vi "make arbitrary waveform_MD.vi"() -> ()   [LabVIEW 2012]
uses:
  Custom Controls/scan mode main settings tab.ctl
  GFG/GFGDisplayRefsGet.vi
  GFG/GFGnumericGet.vi
  GFG/GFGfpRefGet.vi
  GFG/GFGImageRefsGet.vi
  GFG/GFG library.lvlib
  <vilib>/vision/NI_Vision_Development_Module.lvlib
panel:
  out "Source VI":string
  out "error out 3":errorcluster
  out "error out 2":errorcluster
  out "error out":errorcluster
  out "XY Graph 3":cluster{"Y":dbl[], "Y":dbl[]}[](graph)
  out "XY Graph 2":cluster{"Y":dbl[], "Y":dbl[]}[](graph)
  out "XY Graph":cluster{"Y":dbl[], "Y":dbl[]}[](graph)
  out "Waveform Graph 4":dbl[](graph)
  out "Waveform Graph 3":dbl[](graph)
  out "Waveform Graph 2":waveform(dbl)(graph)
  out "Waveform Graph":waveform(dbl)(graph)
  out "size(s) 2":i32
  out "size(s)":i32
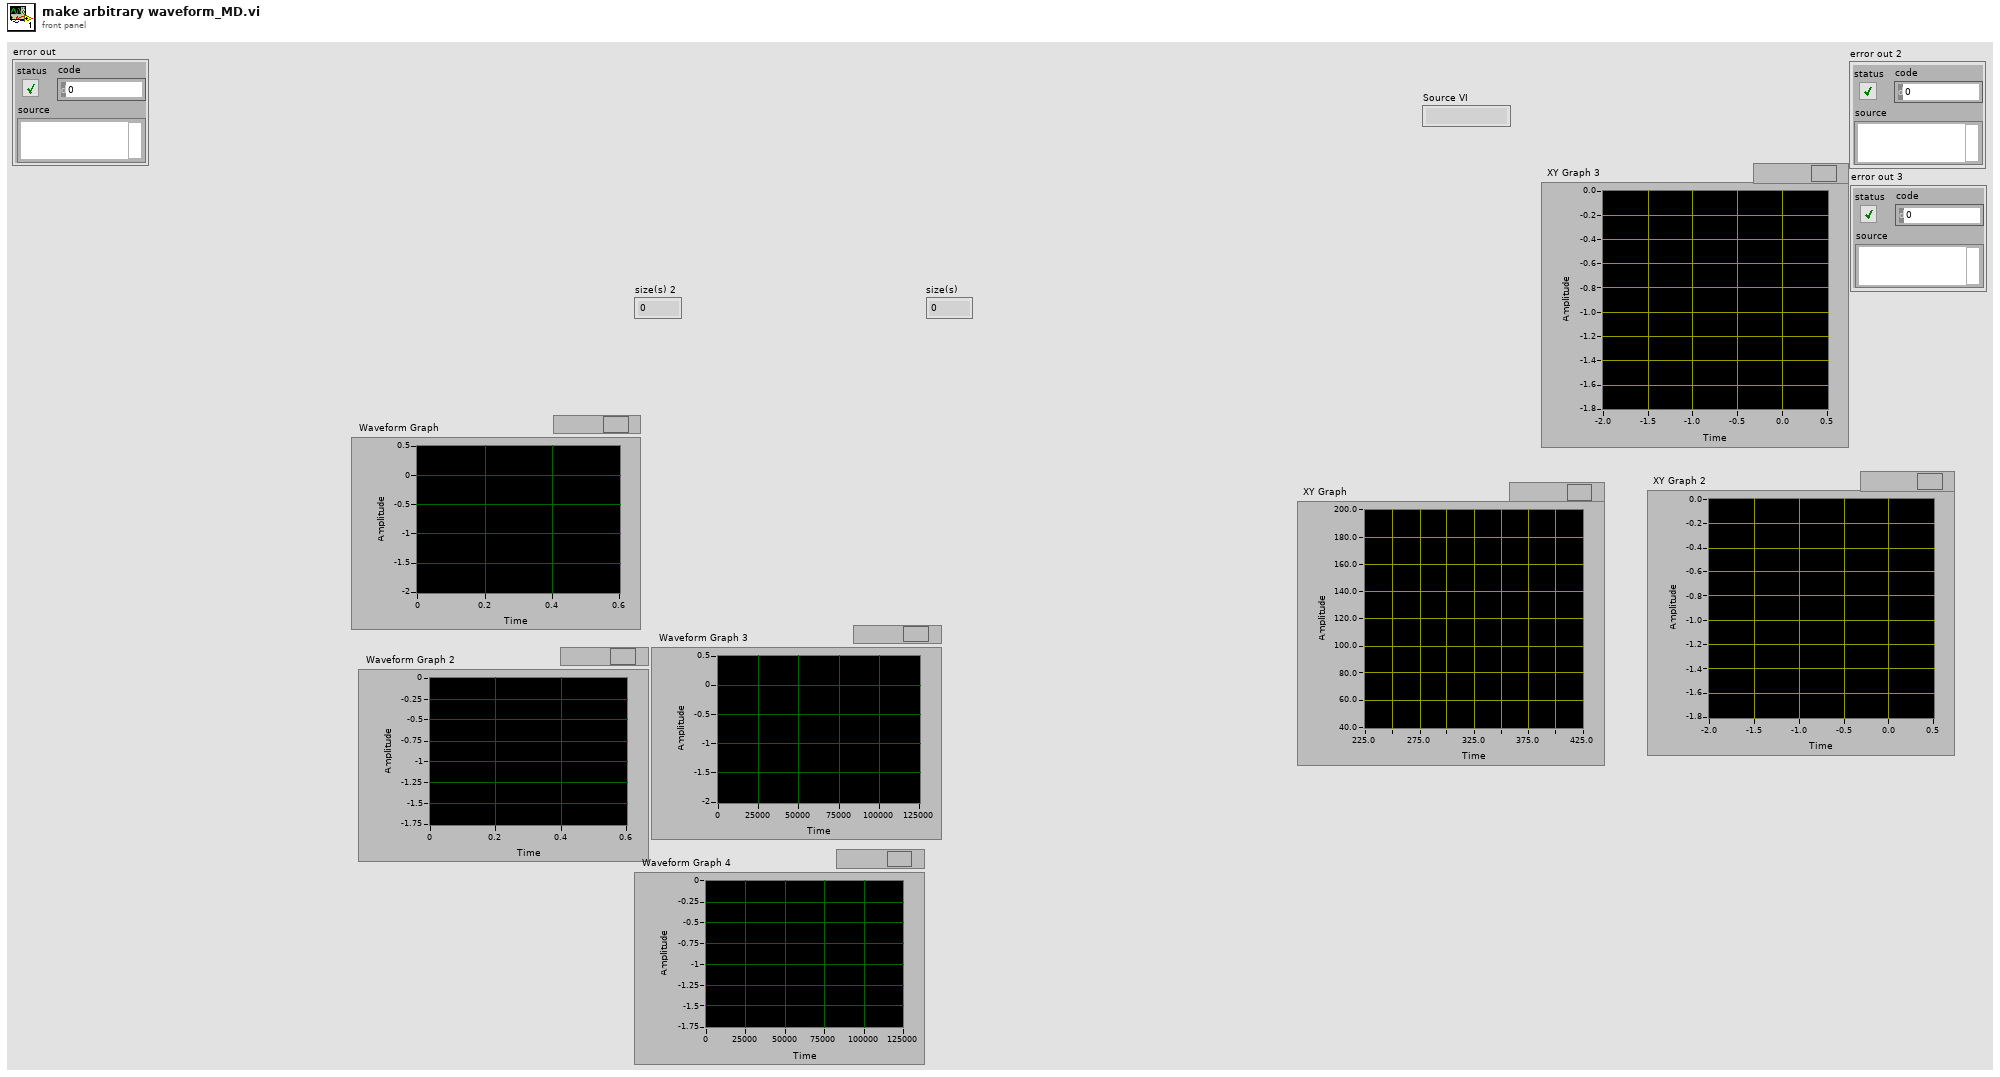
[diagram p1: front panel]
types:
  T1 = cluster{"Channel 1 small":refnum<vi>, "Channel 2 small":refnum<vi>, "Channel 3 small":refnum<vi>, "Channel 4 small":refnum<vi>, "Channel 1 large":refnum<vi>, "Channel 2 large":refnum<vi>, "Channel 3 large":refnum<vi>, "Channel 4 large":refnum<vi>, "RGB overlay":refnum<vi>, "ROI Image display":refnum<vi>, "arb line scan display":refnum<vi>, "Channel 5 large":refnum<vi>}
  T2 = enum8{"Enabled", "Disabled", "Disabled and Grayed Out"}
  T3 = enum32{"Page Enabled", "Page Disabled", "Page Disabled & Grayed"}
  T4 = cluster{"Global Rectangle":i32[], "Contours":cluster{"Contour Type":u32, "ROI Type":u32, "Points":i32[]}[]}
  T5 = typedef "scan mode main settings tab.ctl" = enum32{"2D frame", "2D line scan", "general settings", "Z Stack", "piezo"}
  T6 = typedef "IMAQ Image.ctl" = refnum<image>
  T7 = cluster{"Channel 1 small":T6, "Channel 2 small":T6, "Channel 3 small":T6, "Channel 4 small":T6, "Channel 1 large":T6, "Channel 2 large":T6, "Channel 3 large":T6, "Channel 4 large":T6, "RGB overlay":T6, "ROI Image display":T6, "arb line scan display":T6, "Channel 5 large":T6}
  T8 = cluster{"WaveformChartRef":refnum<vi>, "DigitalRef":refnum<vi>, "ArrayRef":refnum<vi>, "TabControlRef":refnum<vi>, "EnumRef":refnum<vi>, "RingRef":refnum<vi>, "BooleanRef":refnum<vi>, "KnobRef":refnum<vi>, "SlideRef":refnum<vi>, "PathRef":refnum<vi>, "StringRef":refnum<vi>, "ComboBox":refnum<vi>, "WaveformGraphRef":refnum<vi>}
  T9 = typedef "ROI Descriptor" = cluster{"Global Rectangle":i32[], "Contours":cluster{"ID":enum32{"External", "Internal"}, "Type":u32, "Coordinates":i32[]}[]}
  T10 = cluster{"ID":enum32{"External", "Internal"}, "Type":u32, "Coordinates":i32[]}[]
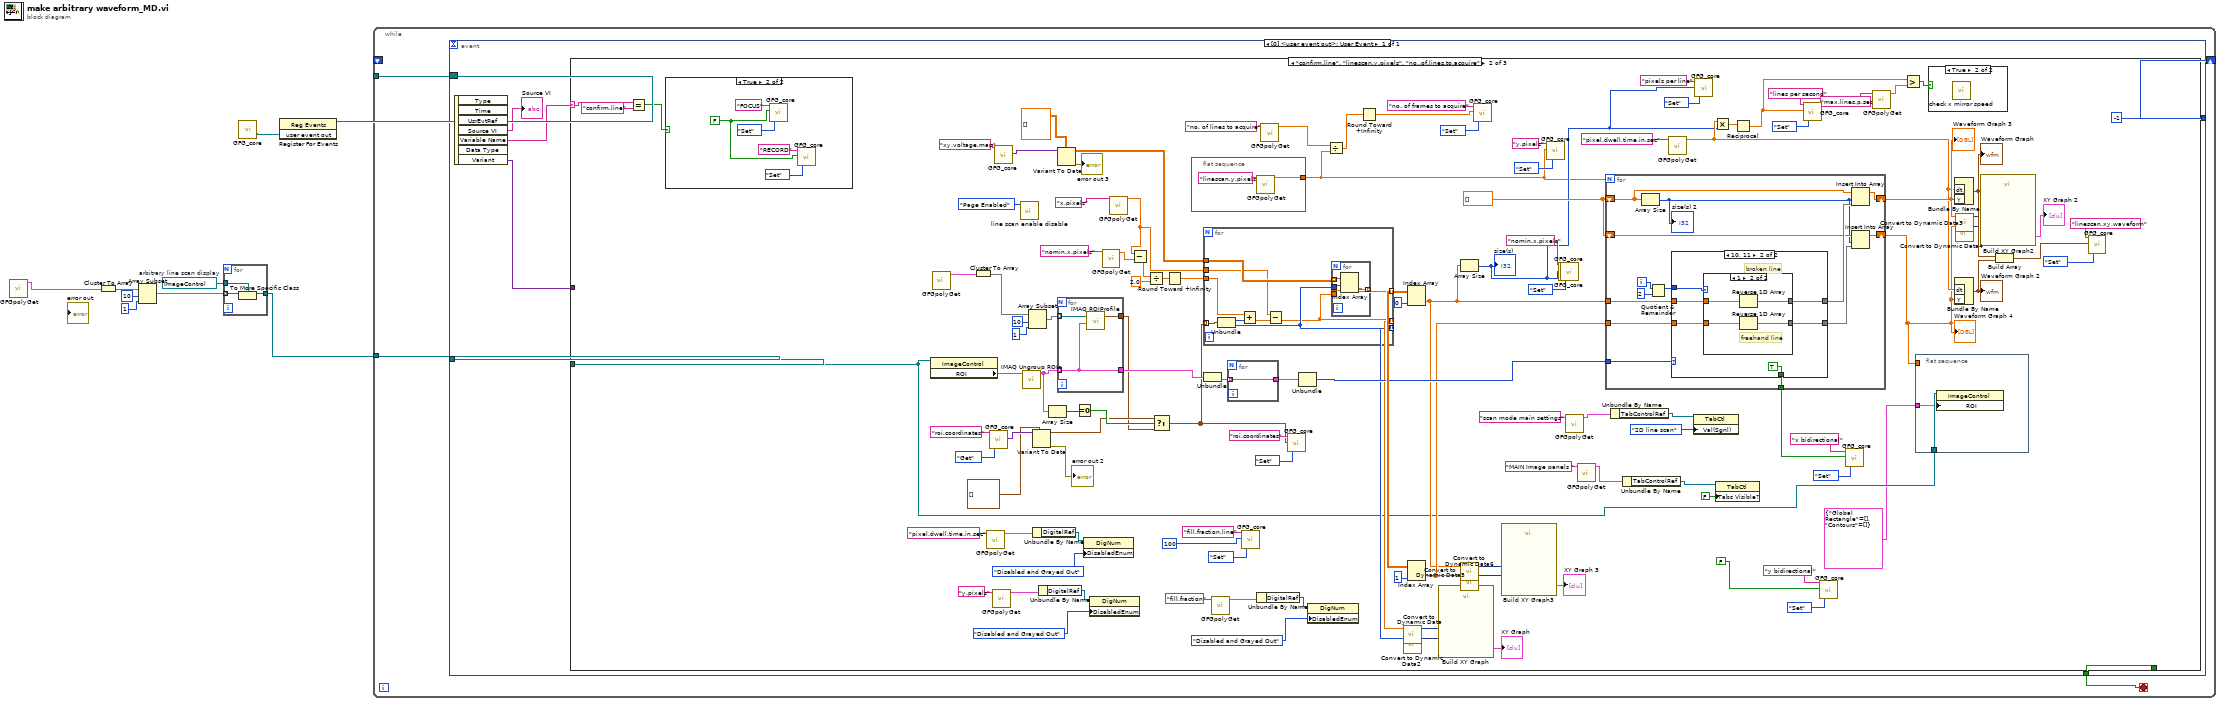
[diagram p0: block diagram]
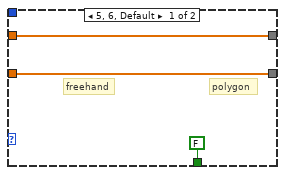
[diagram p5: hidden frame]
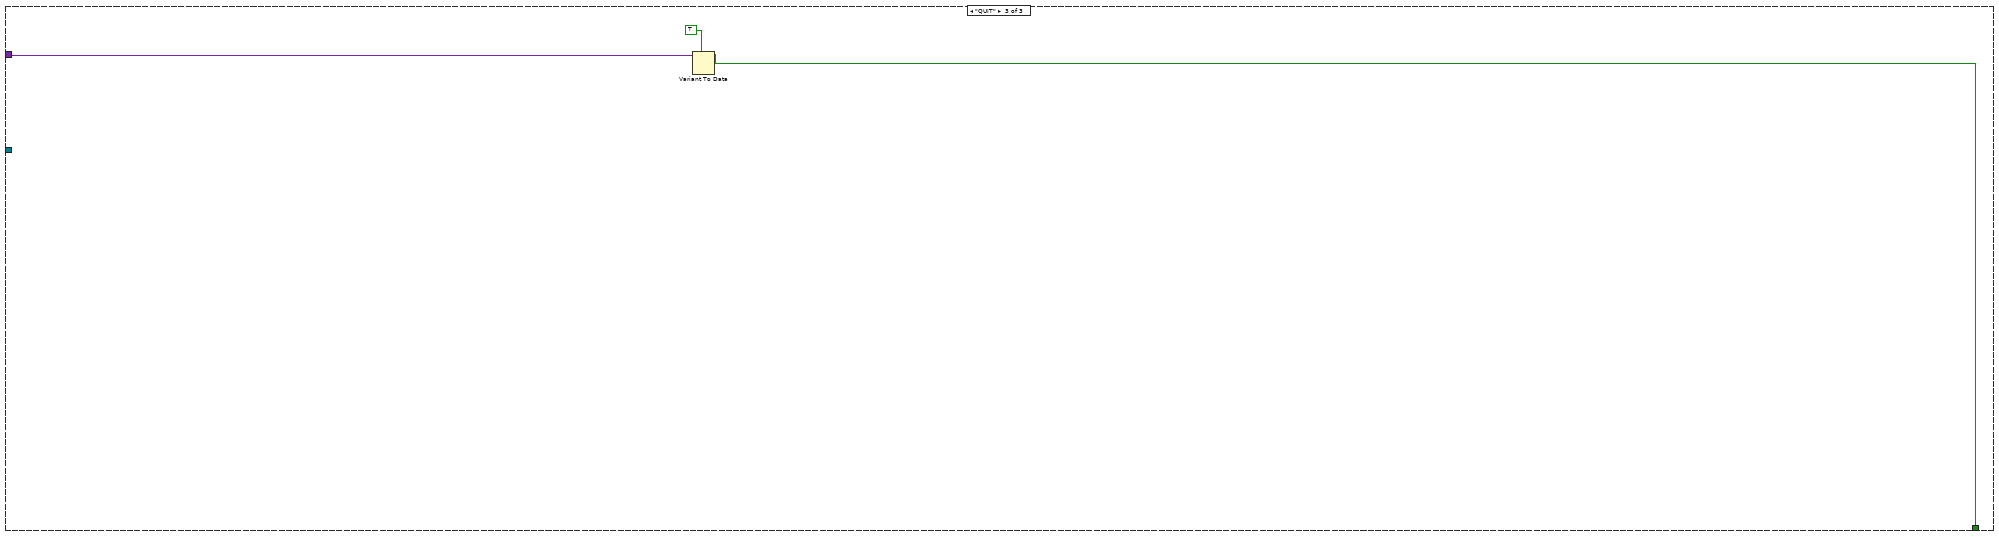
[diagram p7: hidden frame]
diagram:
  w3 = refnum<vi> refnum  # arbitrary line scan display
  n1 = call-poly "GFGpolyGet.vi"() -> ("DisplayRefsOut(generic class)"=w2:T1)  [unwired: 10 in, 1 out]
  n2 = Cluster To Array(cluster=w2) -> (array=w5:refnum<vi>[])
  n3 = Array Subset(array=w5, index=10, length=1) -> (w4:refnum<vi>[])
  n4 = for {
    tunnel: w4 -> [w12] mode=indexing
    tunnel: w3 -> [w11]
    tunnel: [w10] -> w1
    n5 = To More Specific Class(target class=w11, reference=w12) -> (specific class reference=w10:refnum<vi>)  [unwired: 1 in, 1 out]
  }
  n6 = call "GFG_core.vi"() -> ("user event out"=w8:refnum<user-event>)  [unwired: 13 in, 6 out]
  n7 = register-events(w8) -> (reference out=w9:refnum<event-registration>)  [unwired: 2 in, 1 out]
  n8 = while {
    tunnel: w9 -> [w16]
    shift-right: [w14] -> _
    shift-left: _ -> [_]
    tunnel: w1 -> [w13]
    stop <- w15 stop-if-true
    n9 = event shown="[0] <user event out>: User Event" {
      selector: w16 -> [_]
      dyn-events: _ -> [_]
      timeout: _ -> [_]
      tunnel: w13 -> [w22]
      tunnel: [w18] -> w15
      tunnel: [-1 ("length")] -> w14
      event User Event {
        n10 = event-data() -> ("Source VI"=→"Source VI":string, "Variable Name"=w20:string, "Variant"=w19:variant)  [unwired: 1 in, 4 out]
        n11 = case shown="\"confirm.line\", \"linescan.y.pixels\", \"no..of.lines.to.acquire\"" w20 {
          selector: w20 -> [_ w25 _]
          tunnel: w22 -> [_ w76 _]
          tunnel: w19 -> [_ _ w197]
          tunnel: [_ _ w196] -> w18
          frame "False", Default {
          }
          frame "confirm.line", "linescan.y.pixels", "no..of.lines.to.acquire" {
            w119 = dbl[] []
            n12 = Equal?(x=w25, y="confirm.line") -> (x = y?=w23:bool)
            n13 = case shown="True" w23 {
              frame False {
              }
              frame True {
                w141 = FALSE
                n14 = call "GFG_core.vi"("Variable Name in"="FOCUS", "Variant in"=w141, "Action"=enum16{"Init", "Set", "Get"}."Set") -> ()  [unwired: 10 in, 7 out]
                n15 = call "GFG_core.vi"("Variable Name in"="RECORD", "Variant in"=w141, "Action"=enum16{"Init", "Set", "Get"}."Set") -> ()  [unwired: 10 in, 7 out]
              }
            }
            n16 = property class="ImageControl"(reference=w76) -> ("ROI"=w128:T4)  [unwired: 1 in, 2 out]
            n17 = call-poly "GFGpolyGet.vi"() -> ("Image Refs Out"=w139:T7)  [unwired: 10 in, 1 out]
            n18 = Cluster To Array(cluster=w139) -> (array=w138:T6[])
            n19 = call-poly "GFGpolyGet.vi"("Variable Name in"="pixel.dwell.time.in.sec") -> ("output cluster"=w81:T8)  [unwired: 9 in, 1 out]
            n20 = call "GFG_core.vi"("Variable Name in"="roi.coordinates", "Action"=enum16{"Init", "Set", "Get"}."Get") -> ("Variant Out"=w68:variant)  [unwired: 11 in, 6 out]
            n21 = call-poly "GFGpolyGet.vi"("Variable Name in"="y.pixels") -> ("output cluster"=w27:T8)  [unwired: 9 in, 1 out]
            n22 = call "GFG_core.vi"("Variable Name in"="xy.voltage.map") -> ("Variant Out"=w124:variant)  [unwired: 12 in, 6 out]
            n23 = call "line scan enable disable.vi"("Page Enabled State"=T3."Page Enabled") -> ()  [unwired: 11 in]
            n24 = call "IMAQ Ungroup ROIs"("ROI Descriptor"=w128) -> ("ROI Descriptors out"=w70:T9[])  [unwired: 3 in, 1 out]
            n25 = Array Subset(array=w138, index=10, length=1) -> (w134:T6[])
            n26 = Variant To Data(type=cluster{"X":u32, "Y":u32}[] [] ("Pixel Coordinates"), Variant=w68) -> (data=w65:cluster{"X":u32, "Y":u32}[], error out=→"error out 2":errorcluster)  [unwired: 1 in]
            n27 = Unbundle By Name(w81) -> ("DigitalRef"=w82:refnum<vi>)
            n28 = Unbundle By Name(w27) -> ("DigitalRef"=w26:refnum<vi>)
            n29 = Array Size(array=w70) -> (size(s)=w69:i32)
            n30 = for {
              tunnel: w70 -> [w193] mode=indexing
              tunnel: [w193] -> w133
              tunnel: w134 -> [w194] mode=indexing
              tunnel: [w192] -> w64
              n31 = call "IMAQ ROIProfile"("ROI Descriptor"=w193, "Image"=w194) -> ("Pixel Coordinates"=w192:cluster{"X":u32, "Y":u32}[])  [unwired: 2 in, 4 out]
            }
            n32 = Variant To Data(type=dbl[][][] [], Variant=w124) -> (data=w131:dbl[][][], error out=→"error out 3":errorcluster)  [unwired: 1 in]
            n33 = Equal To 0?(x=w69) -> (x = 0?=w66:bool)
            n34 = property class="DigNum"(reference=w82, "DisabledEnum"=T2."Disabled and Grayed Out" ("Disabled")) -> ()  [unwired: 1 in, 2 out]
            n35 = property class="DigNum"(reference=w26, "DisabledEnum"=T2."Disabled and Grayed Out" ("Disabled")) -> ()  [unwired: 1 in, 2 out]
            n36 = call-poly "GFGpolyGet.vi"("Variable Name in"="nomin.x.pixels") -> ("Numeric"=w55:dbl)  [unwired: 9 in, 1 out]
            n37 = call-poly "GFGpolyGet.vi"("Variable Name in"="x.pixels") -> ("Numeric"=w50:dbl)  [unwired: 9 in, 1 out]
            n38 = Subtract(x=w50, y=w55) -> (x-y=w54:dbl)
            n39 = Divide(x=w54, y=2.0) -> (x/y=w52:dbl)
            n40 = Select(t=w65, s=w66, f=w64) -> (s? t:f=w63:cluster{"X":u32, "Y":u32}[])
            n41 = Round Toward +Infinity(x=w52) -> (ceil(x): smallest int >= x=w51:dbl)
            n42 = flat-sequence {
              tunnel: [w146] -> w42
              frame #0 {
                n43 = call-poly "GFGpolyGet.vi"("Variable Name in"="linescan.y.pixels") -> ("Numeric"=w146:dbl)  [unwired: 9 in, 1 out]
              }
            }
            n44 = for {
              tunnel: w63 -> [w187] mode=indexing
              tunnel: [w185] -> w130 mode=indexing
              tunnel: w131 -> [w186]
              tunnel: [w184] -> w126 mode=indexing
              tunnel: [w180] -> w127 mode=indexing
              tunnel: w51 -> [w181]
              tunnel: w50 -> [w179]
              n45 = Unbundle(w187) -> ("X"=w183:u32, "Y"=w184:u32)
              n46 = Add(x=w181, y=w183) -> (x+y=w182:dbl)
              n47 = Subtract(x=w179, y=w182) -> (x-y=w180:dbl)
              n48 = for {
                tunnel: w186 -> [w191] mode=indexing
                tunnel: w180 -> [w190]
                tunnel: w184 -> [w189]
                tunnel: [w188] -> w185 mode=indexing
                n49 = Index Array(array=w191, index (row)=w189, index (col)=w190) -> (element=w188:dbl)
              }
            }
            n50 = Unbundle(w133) -> ("Contours"=w136:T10)  [unwired: 1 out]
            n51 = call-poly "GFGpolyGet.vi"("Variable Name in"="fill.fraction") -> ("output cluster"=w34:T8)  [unwired: 9 in, 1 out]
            n52 = for {
              tunnel: w136 -> [w195] mode=indexing
              tunnel: [w195] -> w135
            }
            n53 = call "GFG_core.vi"("Variable Name in"="fill.fraction.line", "Variant in"=100 ("y"), "Action"=enum16{"Init", "Set", "Get"}."Set") -> ()  [unwired: 10 in, 7 out]
            n54 = Unbundle By Name(w34) -> ("DigitalRef"=w35:refnum<vi>)
            n55 = call-poly "GFGpolyGet.vi"("Variable Name in"="no. of lines to acquire") -> ("Numeric"=w43:dbl)  [unwired: 9 in, 1 out]
            n56 = call "GFG_core.vi"("Variable Name in"="roi.coordinates", "Variant in"=w63, "Action"=enum16{"Init", "Set", "Get"}."Set") -> ()  [unwired: 10 in, 7 out]
            n57 = Unbundle(w135) -> ("Type"=w129:u32)  [unwired: 2 out]
            n58 = property class="DigNum"(reference=w35, "DisabledEnum"=T2."Disabled and Grayed Out" ("Disabled")) -> ()  [unwired: 1 in, 2 out]
            n59 = Divide(x=w43, y=w42) -> (x/y=w41:dbl)
            n60 = Round Toward +Infinity(x=w41) -> (ceil(x): smallest int >= x=w40:dbl)
            n61 = call "Convert to Dynamic Data"("Array"=w127) -> ("Dynamic Data Type"=w117:dynamicdata)  [unwired: 3 in]
            n62 = call "Convert to Dynamic Data2"("Array"=w126) -> ("Dynamic Data Type"=w116:dynamicdata)  [unwired: 3 in]
            n63 = Index Array(array=w130, index (col)=0 ("disabled index (col)")) -> (element=w111:dbl[])  [unwired: 1 in]
            n64 = Index Array(array=w130, index (col)=1 ("disabled index (col)")) -> (element=w112:dbl[])  [unwired: 1 in]
            n65 = call "Build XY Graph"("Y Input"=w116, "X Input"=w117) -> ("XY Graph"=→"XY Graph":cluster{"Y":dbl[], "Y":dbl[]}[])  [unwired: 3 in, 6 out]
            n66 = Array Size(array=w111) -> (size(s)=w47:i32)
            "size(s)" <- w47
            n67 = call "Convert to Dynamic Data5"("Array"=w111) -> ("Dynamic Data Type"=w114:dynamicdata)  [unwired: 3 in]
            n68 = call "Convert to Dynamic Data6"("Array"=w112) -> ("Dynamic Data Type"=w115:dynamicdata)  [unwired: 3 in]
            n69 = call "GFG_core.vi"("Variable Name in"="no. of frames to acquire", "Variant in"=w40, "Action"=enum16{"Init", "Set", "Get"}."Set") -> ()  [unwired: 10 in, 7 out]
            n70 = call "Build XY Graph3"("Y Input"=w115, "X Input"=w114) -> ("XY Graph"=→"XY Graph 3":cluster{"Y":dbl[], "Y":dbl[]}[])  [unwired: 3 in, 6 out]
            n71 = call "GFG_core.vi"("Variable Name in"="y.pixels", "Variant in"=w42, "Action"=enum16{"Init", "Set", "Get"}."Set") -> ()  [unwired: 10 in, 7 out]
            n72 = call "GFG_core.vi"() -> ()  [unwired: 13 in, 7 out]
            n73 = call "GFG_core.vi"("Variable Name in"="nomin.x.pixels", "Variant in"=w47, "Action"=enum16{"Init", "Set", "Get"}."Set") -> ()  [unwired: 10 in, 7 out]
            n74 = call-poly "GFGpolyGet.vi"("Variable Name in"="scan mode main settings") -> ("output cluster"=w90:T8)  [unwired: 9 in, 1 out]
            n75 = call-poly "GFGpolyGet.vi"("Variable Name in"="MAIN Image panels ") -> ("output cluster"=w96:T8)  [unwired: 9 in, 1 out]
            n76 = for {
              N: w42 -> [_]
              tunnel: w112 -> [w161]
              tunnel: w111 -> [w163]
              tunnel: w129 -> [w162]
              shift-right: [w157] -> w101
              shift-left: w119 -> [w152]
              shift-right: [w155] -> w77
              shift-left: w119 -> [w153]
              tunnel: [w150] -> w59
              i -> [w160]
              n77 = Array Size(array=w152) -> (size(s)=w151:i32)
              "size(s) 2" <- w151
              n78 = Quotient & Remainder(x=w160, y=2) -> (x-y*floor(x/y)=w158:i32)  [unwired: 1 out]
              n79 = case shown="10, 11" w162 {
                tunnel: w161 -> [w165 w171]
                tunnel: w163 -> [w166 w172]
                tunnel: [w166 w170] -> w156
                tunnel: [w165 w169] -> w154
                tunnel: w158 -> [_ w168]
                tunnel: [FALSE TRUE] -> w150
                frame 5, 6, Default {
                  # "freehand"
                  # "polygon"
                }
                frame 10, 11 {
                  # "broken line"
                  n80 = case shown="1" w168 {
                    tunnel: w172 -> [w174 w178]
                    tunnel: w171 -> [w173 w177]
                    tunnel: [w174 w176] -> w170
                    tunnel: [w173 w175] -> w169
                    frame 0, Default {
                    }
                    frame 1 {
                      # "freehand line"
                      n81 = Reverse 1D Array(array=w178) -> (reversed array=w176:dbl[])
                      n82 = Reverse 1D Array(array=w177) -> (reversed array=w175:dbl[])
                    }
                  }
                }
              }
              n83 = Insert Into Array(array=w152, index=w151, new element=w156) -> (w157:dbl[])
              n84 = Insert Into Array(array=w153, index=w151, new element=w154) -> (w155:dbl[])
            }
            "Waveform Graph 3" <- w101
            "Waveform Graph 4" <- w77
            n85 = Unbundle By Name(w90) -> ("TabControlRef"=w92:refnum<vi>)
            n86 = Unbundle By Name(w96) -> ("TabControlRef"=w94:refnum<vi>)
            n87 = call-poly "GFGpolyGet.vi"("Variable Name in"="pixel.dwell.time.in.sec" ("Tag in")) -> ("Numeric"=w85:dbl)  [unwired: 9 in, 1 out]
            n88 = property class="TabCtl"(reference=w92, "Val(Sgnl)"=scan_mode_main_settings_tab."2D line scan" ("scan mode main settings")) -> ()  [unwired: 1 in, 2 out]
            n89 = call "GFG_core.vi"("Variable Name in"="pixels per line", "Variant in"=w47, "Action"=enum16{"Init", "Set", "Get"}."Set") -> ()  [unwired: 10 in, 7 out]
            n90 = Multiply(x=w85, y=w47) -> (x*y=w84:dbl)
            n91 = property class="TabCtl"(reference=w94, "Tabs Visible?"=FALSE) -> ()  [unwired: 1 in, 2 out]
            n92 = Reciprocal(x=w84) -> (1/x=w39:dbl)
            n93 = call "GFG_core.vi"("Variable Name in"="lines per second", "Variant in"=w39, "Action"=enum16{"Init", "Set", "Get"}."Set") -> ()  [unwired: 10 in, 7 out]
            n94 = call "GFG_core.vi"("Variable Name in"="y bidirectional", "Variant in"=FALSE, "Action"=enum16{"Init", "Set", "Get"}."Set") -> ()  [unwired: 10 in, 7 out]
            n95 = call "GFG_core.vi"("Variable Name in"="x bidirectional", "Variant in"=w59, "Action"=enum16{"Init", "Set", "Get"}."Set") -> ()  [unwired: 10 in, 7 out]
            n96 = call-poly "GFGpolyGet.vi"("Variable Name in"="max.lines.p.sec") -> ("Numeric"=w37:dbl)  [unwired: 9 in, 1 out]
            n97 = Greater?(x=w39, y=w37) -> (0:w36:bool)
            n98 = flat-sequence {
              tunnel: w77 -> [_]
              tunnel: w76 -> [w149]
              tunnel: T4 {"Global Rectangle"=[], "Contours"=[]} ("ROI") -> [w148]
              frame #0 {
                n99 = property class="ImageControl"(reference=w149, "ROI"=w148) -> ()  [unwired: 1 in, 2 out]
              }
            }
            n100 = case shown="True" w36 {
              frame False {
              }
              frame True {
                n101 = call "check x mirror speed.vi"() -> ()  [unwired: 11 in, 1 out]
              }
            }
            n102 = Bundle By Name("dt"=w85, "Y"=w101) -> (w103:waveform(dbl))  [unwired: 1 in]
            "Waveform Graph" <- w103
            n103 = Bundle By Name("dt"=w85, "Y"=w77) -> (w104:waveform(dbl))  [unwired: 1 in]
            "Waveform Graph 2" <- w104
            n104 = call "Convert to Dynamic Data3"("Array"=w101) -> ("Dynamic Data Type"=w100:dynamicdata)  [unwired: 3 in]
            n105 = call "Convert to Dynamic Data4"("Array"=w77) -> ("Dynamic Data Type"=w99:dynamicdata)  [unwired: 3 in]
            n106 = call "Build XY Graph2"("Y Input"=w99, "X Input"=w100) -> ("XY Graph"=→"XY Graph 2":cluster{"Y":dbl[], "Y":dbl[]}[])  [unwired: 3 in, 6 out]
            n107 = Build Array(w103, w104) -> (w106:waveform(dbl)[])
            n108 = call "GFG_core.vi"("Variable Name in"="linescan.xy.waveform", "Variant in"=w106, "Action"=enum16{"Init", "Set", "Get"}."Set") -> ()  [unwired: 10 in, 7 out]
          }
          frame "QUIT" {
            n109 = Variant To Data(type=TRUE, Variant=w197) -> (data=w196:bool)  [unwired: 1 in, 1 out]
          }
        }
      }
    }
  }
